vi "test_mono_main.vi"(8 "error in":errorcluster) -> (0 "error out":errorcluster)   [LabVIEW 2023, in "horiba.test.lvlib"]
uses:
  horiba.test.lvlib
  Classes/Mono/Monochromator.lvclass
  <vilib>/addons/_JKI Toolkits/Caraya/classes/Test/Test.lvclass
panel:
  # "Connector Pane"
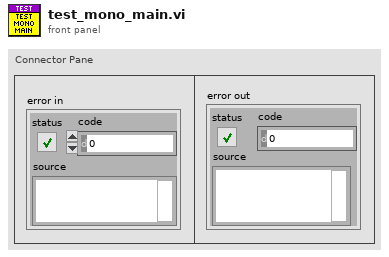
[diagram p1: front panel]
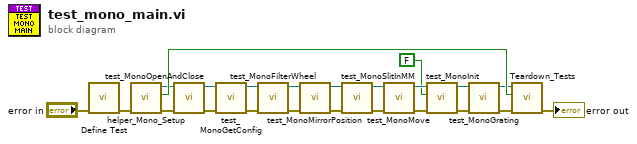
[diagram p0: block diagram]
diagram:
  n1 = call <vilib>:"Define Test.vi"("error in (no error)"="error in") -> ("error out"=w22:errorcluster)  [unwired: 9 in, 1 out]
  n2 = call "helper_Mono_Setup.vi"("error in"=w22) -> ("error out"=w21:errorcluster, "device open for communication?"=w19:bool, "Monochromator out"=w17:refnum<class "Monochromator.lvclass">)  [unwired: 7 in, 1 out]
  n3 = call "test_MonoOpenAndClose.vi"("error in"=w21, "Monochromator in"=w17) -> ("error out"=w18:errorcluster, "Monochromator out"=w16:refnum<class "Monochromator.lvclass">)  [unwired: 8 in]
  n4 = call "test_MonoGetConfig.vi"("error in"=w18, "Monochromator in"=w16) -> ("error out"=w15:errorcluster, "Monochromator out"=w14:refnum<class "Monochromator.lvclass">)  [unwired: 8 in]
  n5 = call "test_MonoFilterWheel.vi"("error in"=w15, "Monochromator in"=w14) -> ("error out"=w13:errorcluster, "Monochromator out"=w12:refnum<class "Monochromator.lvclass">)  [unwired: 8 in]
  n6 = call "test_MonoMirrorPosition.vi"("error in"=w13, "Monochromator in"=w12) -> ("error out"=w11:errorcluster, "Monochromator out"=w10:refnum<class "Monochromator.lvclass">)  [unwired: 8 in]
  n7 = call "test_MonoSlitInMM.vi"("error in"=w11, "Monochromator in"=w10) -> ("error out"=w8:errorcluster, "Monochromator out"=w9:refnum<class "Monochromator.lvclass">)  [unwired: 8 in]
  n8 = call "test_MonoMove.vi"("error in"=w8, "Monochromator in"=w9) -> ("error out"=w6:errorcluster, "Monochromator out"=w7:refnum<class "Monochromator.lvclass">)  [unwired: 8 in]
  n9 = call "test_MonoInit.vi"("error in"=w6, "force"=FALSE, "Monochromator in"=w7) -> ("error out"=w4:errorcluster, "Monochromator out"=w3:refnum<class "Monochromator.lvclass">)  [unwired: 6 in, 1 out]
  n10 = call "test_MonoGrating.vi"("error in"=w4, "Monochromator in"=w3) -> ("error out"=w2:errorcluster, "Monochromator out"=w1:refnum<class "Monochromator.lvclass">)  [unwired: 7 in, 1 out]
  n11 = call "Teardown_Tests.vi"("error in"=w2, "Module Was Already Running?"=w19, "horiba.lvlib:GenericDevice"=w1) -> ("error out"=→"error out":errorcluster)  [unwired: 7 in, 1 out]
